vi "Blynk Email.vi"(6 "message":string, 8 "error in (no error)":errorcluster, 9 "topic":string, 10 "to":string, 11 "connection":refnum<k5>) -> (0 "error out":errorcluster, 3 "connection out":refnum<k5>)   [LabVIEW 2014]
uses:
  utilities/MsgType.ctl
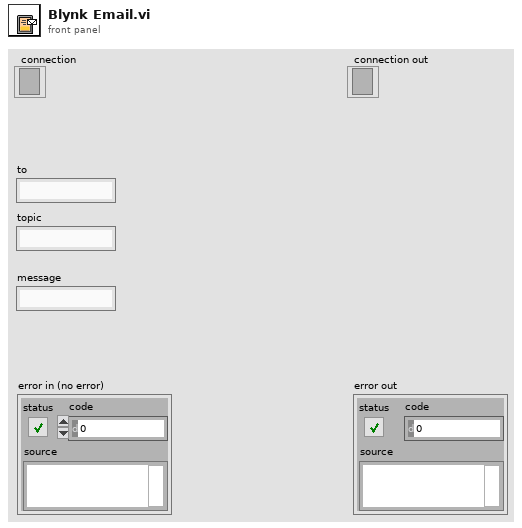
[diagram p1: front panel]
types:
  T1 = typedef "MsgType.ctl" = enum8{"RSP", "REGISTER", "LOGIN", "SAVE_PROF", "LOAD_PROF", "GET_TOKEN", "PING", "ACTIVATE", "DEACTIVATE", "REFRESH", "UNDEFINED0", "UNDEFINED1", "TWEET", "EMAIL", "NOTIFY", "BRIDGE", "UNDEFINED2", "UNDEFINED3", "UNDEFINED4", "UNDEFINED5", "HW"}
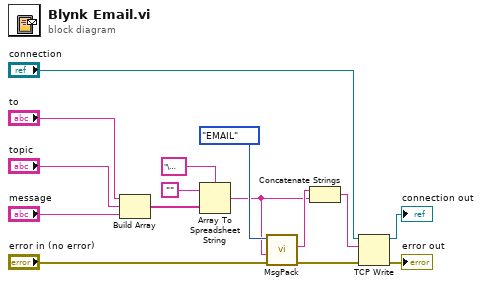
[diagram p0: block diagram]
diagram:
  n1 = Build Array("to", "topic", "message") -> (w5:string[])
  n2 = Array To Spreadsheet String(delimiter (Tab)="\u0000", array=w5, 3:"") -> (spreadsheet string=w11:string)
  n3 = call "MsgPack.vi"("error in"="error in (no error)", "msg"=w11, "msg_type"=MsgType."EMAIL") -> ("error out"=w1:errorcluster, "msg_data"=w14:string)  [unwired: 7 in]
  n4 = Concatenate Strings(w14, w11) -> (w15:string)
  n5 = TCP Write(connection ID="connection", data in=w15, error in (no error)=w1) -> (connection ID out=→"connection out":refnum<k5>, error out=→"error out":errorcluster)  [unwired: 1 in, 1 out]
